vi "DIO Set.vi"(7 "Box ID":u8=1, 8 "error in (no error)":errorcluster, 9 "DIO Enable":bool[](array[boolean]), 10 "DIO Direction":bool[](array[boolean]), 11 "CAN in":refnum<class "XNET_BS120x.lvclass">) -> (0 "error out":errorcluster, 3 "CAN out":refnum<class "XNET_BS120x.lvclass">)   [LabVIEW 2021, in "BS120x Driver.lvlib" / "XNET_BS120x.lvclass"]
uses:
  XNET_BS120x.lvclass
  BS120x.lvclass
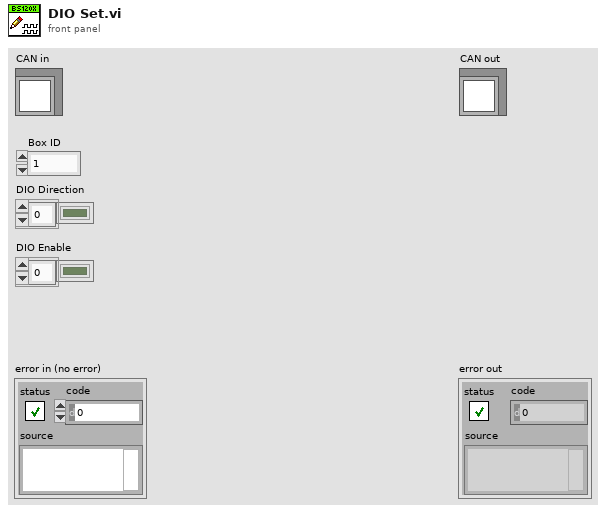
[diagram p1: front panel]
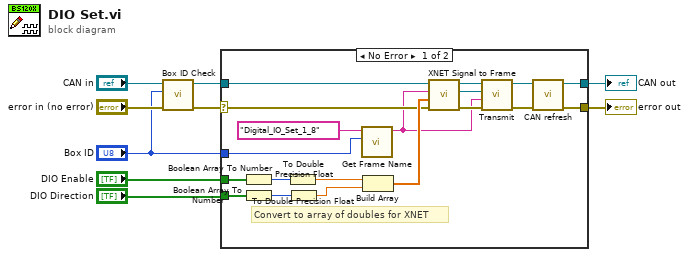
[diagram p0: block diagram]
diagram:
  n1 = call "Box ID Check.vi"("error in (no error)"="error in (no error)", "Box ID"="Box ID", "CAN in"="CAN in") -> ("error out"=w5:errorcluster, "CAN out"=w6:refnum<class "XNET_BS120x.lvclass">)  [unwired: 7 in]
  n2 = case shown="No Error" w5 {
    selector: w5 -> [w11 w29]
    tunnel: "DIO Enable" -> [w24 _]
    tunnel: "DIO Direction" -> [w23 _]
    tunnel: w6 -> [w20 w30]
    tunnel: [w16 w29] -> w8
    tunnel: [w14 w30] -> w7
    tunnel: "Box ID" -> [w12 _]
    frame No Error {
      # "Convert to array of doubles for XNET"
      n3 = Boolean Array To Number(Boolean array=w24) -> (number=w27:u32)
      n4 = Boolean Array To Number(Boolean array=w23) -> (number=w28:u32)
      n5 = To Double Precision Float(number=w27) -> (double precision float=w26:dbl)
      n6 = To Double Precision Float(number=w28) -> (double precision float=w25:dbl)
      n7 = call "Get Frame Name.vi"("Box ID"=w12, "Frame Name"="Digital_IO_Set_1_8" ("Frame")) -> ("Frame Name out"=w10:string)  [unwired: 9 in]
      n8 = Build Array(w26, w25) -> (w21:dbl[])
      n9 = call "XNET Signal to Frame.vi"("error in (no error)"=w11, "Data Array"=w21, "Frame"=w10, "CAN in"=w20) -> ("error out"=w22:errorcluster, "Data"=w18:refnum<class "XNET Data.lvclass">, "CAN out"=w19:refnum<class "XNET_BS120x.lvclass">)  [unwired: 5 in]
      n10 = call "Transmit.vi"("error in (no error)"=w22, "Frame"=w10, "Data in"=w18, "CAN in"=w19) -> ("error out"=w17:errorcluster, "CAN out"=w15:refnum<class "XNET_BS120x.lvclass">)  [unwired: 6 in]
      n11 = call "CAN refresh.vi"("error in (no error)"=w17, "CAN in"=w15) -> ("error out"=w16:errorcluster, "CAN out"=w14:refnum<class "XNET_BS120x.lvclass">)  [unwired: 8 in]
    }
    frame Error {
    }
  }
  "error out" <- w8
  "CAN out" <- w7
